vi "Stop.vi"(8 "error in (no error)":errorcluster, 11 "PID Loop in":refnum<class "PID Loop.lvclass">) -> (3 "PID Loop out":refnum<class "PID Loop.lvclass">)   [LabVIEW 2024, in "PID Loop.lvlib" / "PID Loop.lvclass"]
uses:
  PID Loop.lvclass
  PID Loop.lvclass/PID Loop.ctl
  src/Zero Timeout Message Handler/Zero Timeout Message Handler/Zero Timeout Message Handler.lvclass
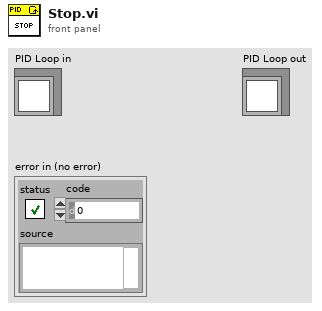
[diagram p1: front panel]
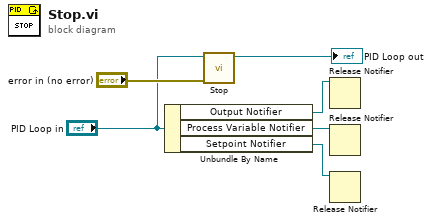
[diagram p0: block diagram]
diagram:
  n1 = Unbundle By Name("PID Loop in") -> ("Output Notifier"=w3:refnum<notifier>, "Process Variable Notifier"=w2:refnum<notifier>, "Setpoint Notifier"=w1:refnum<notifier>)
  n2 = call-parent "Stop.vi"("error in (no error)"="error in (no error)", "Zero Timeout Message Handler in"="PID Loop in") -> ("Zero Timeout Message Handler out"=→"PID Loop out":refnum<class "PID Loop.lvclass">)  [unwired: 9 in]
  n3 = Release Notifier(notifier=w3) -> ()  [unwired: 2 in, 3 out]
  n4 = Release Notifier(notifier=w2) -> ()  [unwired: 2 in, 3 out]
  n5 = Release Notifier(notifier=w1) -> ()  [unwired: 2 in, 3 out]
